vi "UserMgt.vi"(11 "UserLibFile":path=path "d:/test.usr") -> ()   [LabVIEW 2020]
panel:
  in  "Group:":u8(ring) items=["Operator", "Engineering", "Admin"]
  in  "Pwd":string caption="Password:"
  in  "User":string caption="User Name:"
  in  "Delete":bool
  in  "Exit":bool
  in  "Add":bool
  in  "Users":i32(listbox)
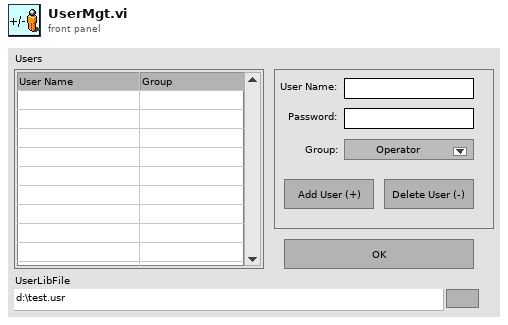
[diagram p1: front panel]
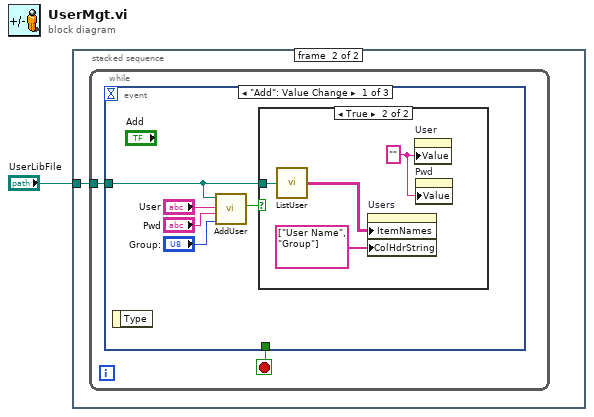
[diagram p0: block diagram]
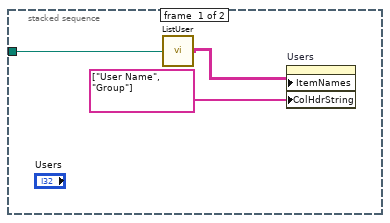
[diagram p2: hidden frame]
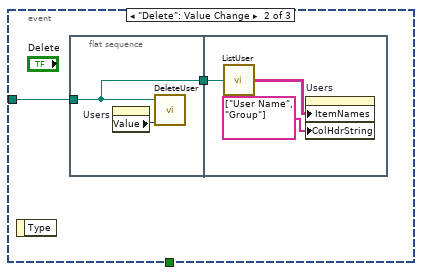
[diagram p4: hidden frame]
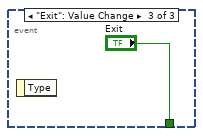
[diagram p5: hidden frame]
diagram:
  n1 = stacked-sequence {
    tunnel: "UserLibFile" -> [w2 w5]
    frame #0 {
      n2 = call "ListUser.vi"("UserLibFile"=w2) -> ("Users"=w3:string[][])
      n3 = property on="Users" class="MCListbox (strict)"("ItemNames"=w3, "ColHdrString"=string[] ["User Name", "Group"] ("Column Header Strings[]")) -> ()  [unwired: 2 in, 2 out]
    }
    frame #1 {
      n4 = while {
        tunnel: w5 -> [w6]
        stop <- w7 stop-if-true
        n5 = event shown="[0] \"Add\": Value Change" {
          selector: _ -> [_ _ _]
          dyn-events: _ -> [_ _ _]
          timeout: _ -> [_ _ _]
          tunnel: [_ _ "Exit"] -> w7
          tunnel: w6 -> [w8 w18 _]
          event "Add": Value Change {
            n6 = event-data() -> ()  [unwired: 2 out]
            n7 = call "AddUser.vi"("Group"="Group:", "Pwd"="Pwd", "User"="User", "UserLibFile"=w8) -> ("Success?"=w11:bool)  [unwired: 7 in]
            n8 = case shown="True" w11 {
              tunnel: w8 -> [_ w13]
              frame False {
              }
              frame True {
                w16 = "" ("User")
                n9 = call "ListUser.vi"("UserLibFile"=w13) -> ("Users"=w14:string[][])
                n10 = property on="Users" class="MCListbox (strict)"("ItemNames"=w14, "ColHdrString"=string[] ["User Name", "Group"] ("Column Header Strings[]")) -> ()  [unwired: 2 in, 2 out]
                n11 = property on="User" class="Str"("Value"=w16) -> ()  [unwired: 2 in, 2 out]
                n12 = property on="Pwd" class="Str"("Value"=w16) -> ()  [unwired: 2 in, 2 out]
              }
            }
          }
          event "Delete": Value Change {
            n13 = event-data() -> ()  [unwired: 2 out]
            n14 = flat-sequence {
              tunnel: w18 -> [w19]
              tunnel: [w19] -> w17
              tunnel: w17 -> [w21]
              frame #0 {
                n15 = property on="Users" class="MCListbox (strict)"() -> ("Value"=w20:i32)  [unwired: 2 in, 2 out]
                n16 = call "DeleteUser.vi"("index"=w20, "UserLibFile"=w19) -> ()  [unwired: 10 in]
              }
              frame #1 {
                n17 = call "ListUser.vi"("UserLibFile"=w21) -> ("Users"=w23:string[][])
                n18 = property on="Users" class="MCListbox (strict)"("ItemNames"=w23, "ColHdrString"=string[] ["User Name", "Group"] ("Column Header Strings[]")) -> ()  [unwired: 2 in, 2 out]
              }
            }
          }
          event "Exit": Value Change {
            n19 = event-data() -> ()  [unwired: 2 out]
          }
        }
      }
    }
  }
